vi "AddPersonnel.vi"(8 "error in (no error)":errorcluster, 10 "Personnel":string, 11 "Room Number":i32) -> (0 "error out":errorcluster, 2 "Response":string)   [LabVIEW 2015, in "RoomRestApi.lvlib"]
uses:
  RoomRestApi.lvlib
  TypeDef/PostRoomCommands.ctl
panel:
  out "JSON string":string
  # "{\"FlagsState\":\"{\\\"State\\\":[false,false,false,false],\\\"Color\\\":[0,1,2,3]}\"}"
  # "http://127.0.0.1:8001/WebService1/UpdateFlagState?Room={value}&FlagState={value}"
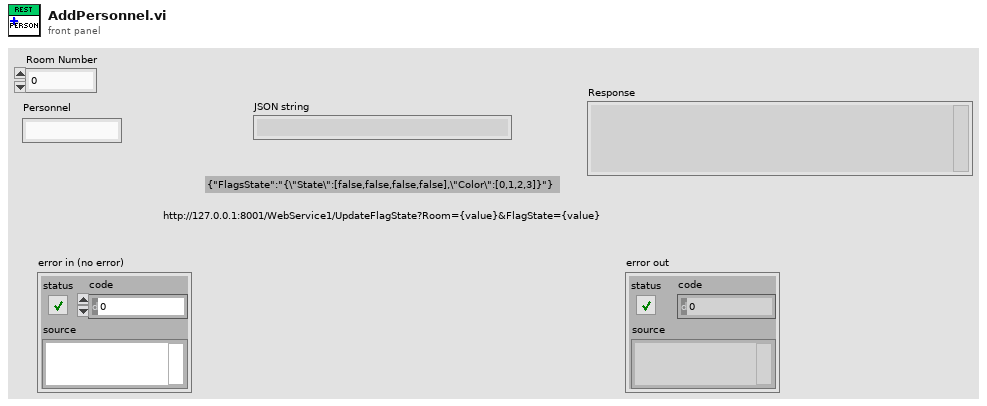
[diagram p1: front panel]
types:
  T1 = typedef "RoomRestApi.lvlib/PostRoomCommands.ctl" = enum16{"WriteFlagState", "WriteFlagColor", "WriteBedVacant", "AddPersonnel", "RemovePersonnel", "AddRequest", "RemoveRequest", "WriteBeaconID", "WriteBedURL", "WriteFlag"}
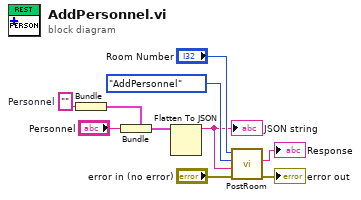
[diagram p0: block diagram]
diagram:
  w1 = ""  # Personnel
  n1 = Bundle("Personnel"=w1) -> (w4:cluster{"Personnel":string})  [unwired: 1 in]
  n2 = Bundle(cluster=w4, "Personnel"="Personnel") -> (w3:cluster{"Personnel":string})
  n3 = Flatten To JSON(anything=w3) -> (JSON string=w5:string)  [unwired: 2 in, 1 out]
  "JSON string" <- w5
  n4 = call "PostRoom.vi"("error in (no error)"="error in (no error)", "Data"=w5, "Commands"=PostRoomCommands."AddPersonnel" ("Enum"), "Room Number"="Room Number") -> ("error out"=→"error out":errorcluster, "body"=→"Response":string)  [unwired: 6 in]
